vi "Logitech F310.vi"(0 "refnum name":string, 1 "error in (no error)":errorcluster) -> (2 "error out":errorcluster, 3 "D-Pad Buttons":T1, 4 "Left Stick":cluster{"X":dbl, "Y":dbl}, 5 "Right Stick":cluster{"X":dbl, "Y":dbl}, 6 "D-Pad":cluster{"X":dbl, "Y":dbl}, 7 "Buttons":T2)   [LabVIEW 2013]
uses:
  <vilib>/Rock Robotics/WPI/Joystick/WPI_JoystickGetSetRefNum.vi
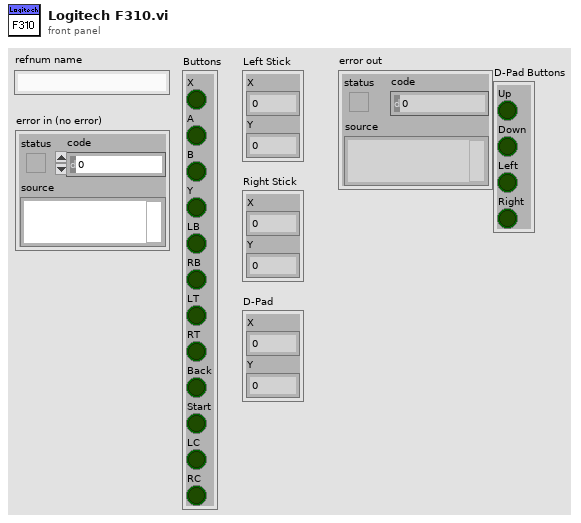
[diagram p1: front panel]
types:
  T1 = cluster{"Up":bool, "Down":bool, "Left":bool, "Right":bool}
  T2 = cluster{"X":bool, "A":bool, "B":bool, "Y":bool, "LB":bool, "RB":bool, "LT":bool, "RT":bool, "Back":bool, "Start":bool, "LC":bool, "RC":bool}
  T3 = typedef "WPI_JoystickDevRef.ctl" = cluster{"Device":T4}
  T4 = typedef "WPI_JoystickDeviceEnum.ctl" = enum16{"USB 1", "USB 2", "USB 3", "USB 4", "Kinect 1", "Kinect 2"}
  T5 = typedef "WPI_JoystickButtonState.ctl" = cluster{"Button 1":bool, "Button 2":bool, "Button 3":bool, "Button 4":bool, "Button 5":bool, "Button 6":bool, "Button 7":bool, "Button 8":bool, "Button 9":bool, "Button 10":bool, "Button 11":bool, "Button 12":bool}
  T6 = cluster{"axis 1 (x)":dbl, "axis 2 (y)":dbl, "axis 3 (throttle)":dbl, "axis 4":dbl, "axis 5":dbl, "axis 6":dbl}
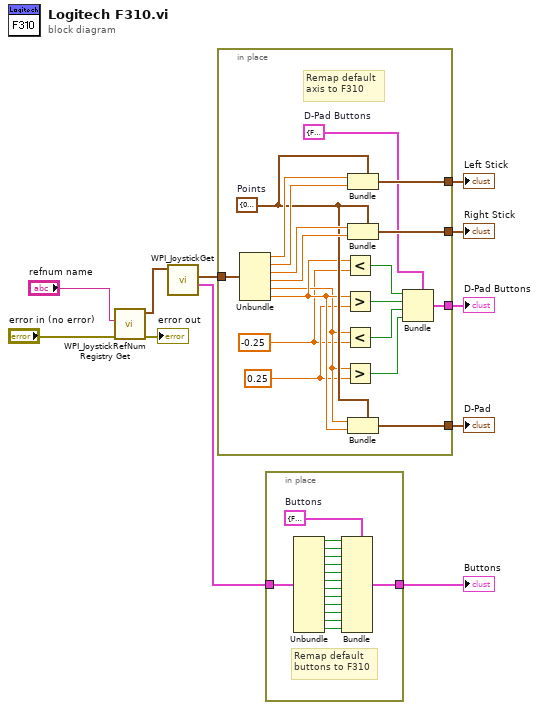
[diagram p0: block diagram]
diagram:
  n1 = call <vilib>:"WPI_JoystickRefNum Registry Get.vi"("error in (no error)"="error in (no error)", "refnum name"="refnum name") -> ("error out"=→"error out":errorcluster, "JoystickDevRef"=w11:T3)  [unwired: 8 in]
  n2 = call <vilib>:"WPI_JoystickGet.vi"("JoystickDevRef"=w11) -> ("Buttons"=w9:T5, "Axes"=w10:T6)  [unwired: 4 in, 1 out]
  n3 = in-place {
    in-place-border: w10 -> [w30]
    in-place-border: [w25] -> w5
    in-place-border: [w24] -> w4
    in-place-border: [w22] -> w3
    in-place-border: [w16] -> w1
    w17 = -0.25 ("y")
    w18 = 0.25 ("y")
    w21 = T1 {"Up"=FALSE, "Down"=FALSE, "Left"=FALSE, "Right"=FALSE}  # D-Pad Buttons
    w23 = cluster{"X":dbl, "Y":dbl} {"X"=0.0, "Y"=0.0}  # Points
    # "Remap default\naxis to F310"
    n4 = Unbundle(w30) -> ("axis 1 (x)"=w29:dbl, "axis 2 (y)"=w28:dbl, "axis 3 (throttle)"=w27:dbl, "axis 4"=w26:dbl, "axis 5"=w19:dbl, "axis 6"=w20:dbl)
    n5 = Less?(x=w20, y=w17) -> (x < y?=w14:bool)
    n6 = Greater?(x=w20, y=w18) -> (0:w15:bool)
    n7 = Less?(x=w19, y=w17) -> (x < y?=w12:bool)
    n8 = Greater?(x=w19, y=w18) -> (0:w13:bool)
    n9 = Bundle(cluster=w23, "X"=w29, "Y"=w28) -> (w25:cluster{"X":dbl, "Y":dbl})
    n10 = Bundle(cluster=w23, "X"=w27, "Y"=w26) -> (w24:cluster{"X":dbl, "Y":dbl})
    n11 = Bundle(cluster=w23, "X"=w19, "Y"=w20) -> (w22:cluster{"X":dbl, "Y":dbl})
    n12 = Bundle(cluster=w21, "Up"=w14, "Down"=w15, "Left"=w12, "Right"=w13) -> (w16:T1)
  }
  "Left Stick" <- w5
  "Right Stick" <- w4
  "D-Pad" <- w3
  "D-Pad Buttons" <- w1
  n13 = in-place {
    in-place-border: w9 -> [w45]
    in-place-border: [w31] -> w2
    w44 = T2 {"X"=FALSE, "A"=FALSE, "B"=FALSE, "Y"=FALSE, "LB"=FALSE, "RB"=FALSE, "LT"=FALSE, "RT"=FALSE, "Back"=FALSE, "Start"=FALSE, "LC"=FALSE, "RC"=FALSE}  # Buttons
    # "Remap default\nbuttons to F310"
    n14 = Unbundle(w45) -> ("Button 1"=w43:bool, "Button 2"=w42:bool, "Button 3"=w41:bool, "Button 4"=w40:bool, "Button 5"=w39:bool, "Button 6"=w38:bool, "Button 7"=w37:bool, "Button 8"=w36:bool, "Button 9"=w35:bool, "Button 10"=w34:bool, "Button 11"=w33:bool, "Button 12"=w32:bool)
    n15 = Bundle(cluster=w44, "X"=w43, "A"=w42, "B"=w41, "Y"=w40, "LB"=w39, "RB"=w38, "LT"=w37, "RT"=w36, "Back"=w35, "Start"=w34, "LC"=w33, "RC"=w32) -> (w31:T2)
  }
  "Buttons" <- w2
